vi "motorPwm.vi"(7 "reverse?":bool, 8 "error in (no error)":errorcluster, 10 "Speed (PWM)":dbl) -> (0 "error out":errorcluster)   [LabVIEW 2019, in "SJCube_KNRm.lvlib"]
uses:
  SJCube_KNRm.lvlib
  KNRm_ReMi_OS5.lvlibp
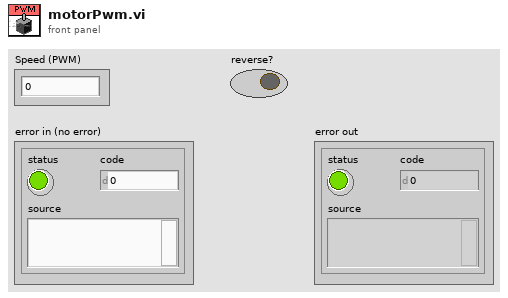
[diagram p1: front panel]
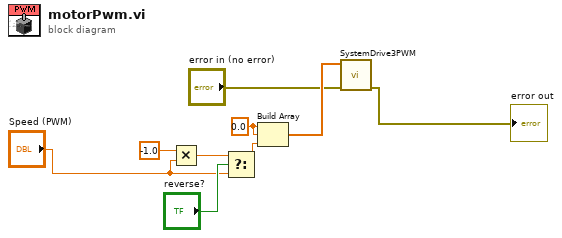
[diagram p0: block diagram]
diagram:
  w4 = 0.0 ("element")
  n1 = Multiply(x=-1.0, y="Speed (PWM)") -> (x*y=w8:dbl)
  n2 = Select(t=w8, s="reverse?", f="Speed (PWM)") -> (s? t:f=w5:dbl)
  n3 = Build Array(w4, w4, w5) -> (w3:dbl[])
  n4 = call "SystemDrive3PWM.vi"("error in"="error in (no error)", "3xMotorSpeed(PWM%)"=w3) -> ("error out"=→"error out":errorcluster)  [unwired: 8 in, 1 out]
